vi "FTW-Container-Object-DeleteAllElements.vi"(0 "FTW-Container In":refnum<class "FTW-Container.lvclass">, 11 "error in":errorcluster) -> (4 "FTW-Container Out":refnum<class "FTW-Container.lvclass">, 15 "error out":errorcluster)   [LabVIEW 2015, in "FTW-Container.lvclass"]
uses:
  FTW-Container.lvclass
  FTW-Container.lvclass/FTW-Container.ctl
  <vilib>/Utility/Data Type/NI_Data Type.lvlib
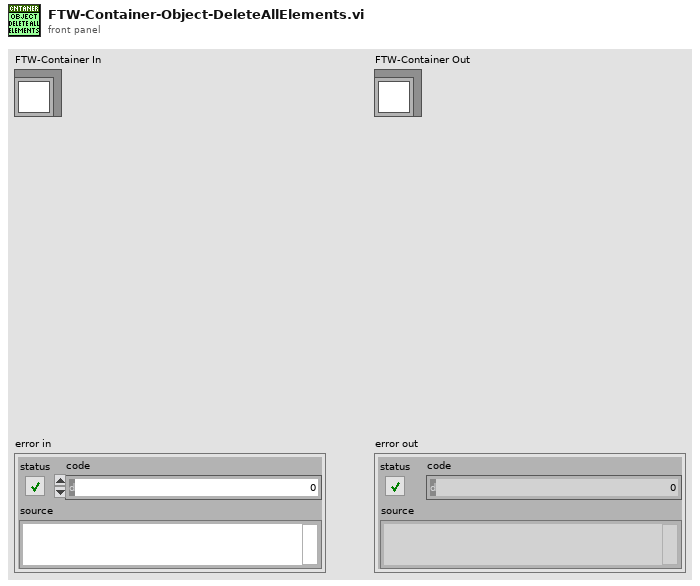
[diagram p1: front panel]
types:
  T1 = typedef "NI_Data Type.lvlib/Data Type.ctl" = enum8{"Invalid Type", "Void", "I8", "I16", "I32", "I64", "U8", "U16", "U32", "U64", "Single Float", "Double Float", "Extended Float", "Single Complex", "Double Complex", "Extended Complex", "Enum U8", "Enum U16", "Enum U32", "Enum U64", "Single Float With Unit", "Double Float With Unit", "Extended Float With Unit", "Single Complex with Unit", "Double Complex with Unit", "Extended Complex with Unit", "Boolean", "String", "Path", "Picture", "Tag", "Array", "Cluster", "Variant", "LV Variant", "Waveform", "Timestamp", "Digital Waveform", "Digital Data", "ExpressData", "Refnum", "External Data", "VI", "Poly VI", "LabVIEW Class Instance", "Fixed Point"}
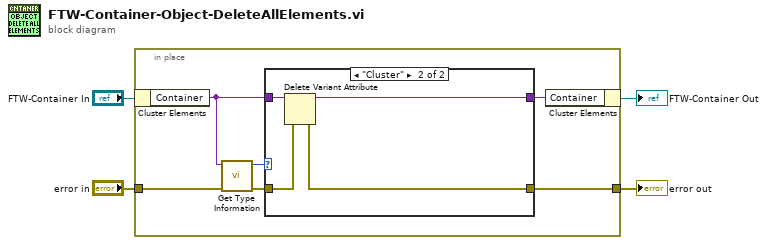
[diagram p0: block diagram]
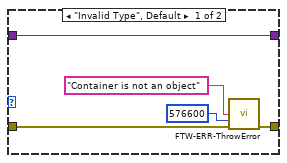
[diagram p2: hidden frame]
diagram:
  n1 = in-place {
    in-place-border: "error in" -> [w10]
    in-place-border: [w8] -> w3
    n2 = in-place-cluster #1("FTW-Container In") -> ("Container"=w6:variant)
    n3 = call <vilib>:"Get Type Information.vi"("error in (no error)"=w10, "Variant"=w6) -> ("error out"=w9:errorcluster, "Type"=w7:T1)  [unwired: 5 in, 3 out]
    n4 = case shown="\"Cluster\"" w7 {
      tunnel: w9 -> [w15 w19]
      tunnel: [w14 w17] -> w8
      tunnel: w6 -> [w11 w18]
      tunnel: [w11 w16] -> w5
      frame "Invalid Type", Default {
        n5 = call "FTW-ERR-ThrowError.vi"("Error Message"="Container is not an object", "Error Code"=576600, "error in"=w15) -> ("error out"=w14:errorcluster)  [unwired: 12 in]
      }
      frame "Cluster" {
        n6 = Delete Variant Attribute(4:w19, 7:w18) -> (0:w17:errorcluster, 3:w16:variant)  [unwired: 1 in, 1 out]
      }
    }
    n7 = in-place-cluster #1("Container"=w5) -> (→"FTW-Container Out":refnum<class "FTW-Container.lvclass">)
  }
  "error out" <- w3
